vi "LCR_Readout.vi"(8 "error in (no error)":errorcluster, 11 "WK6440B in":refnum<class "WK6440B.lvclass">) -> (0 "error out":errorcluster, 1 "Resistance in Ohm":dbl, 2 "Capacitance in pF":dbl, 3 "WK6440B out":refnum<class "WK6440B.lvclass">)   [LabVIEW 2018, in "WK6440B.lvclass"]
uses:
  WK6440B.lvclass
  F:/itk-strip-sensor-qc/LabVIEW 2013/InstrControl/InstrControl.lvclass
  InstrControl.lvclass
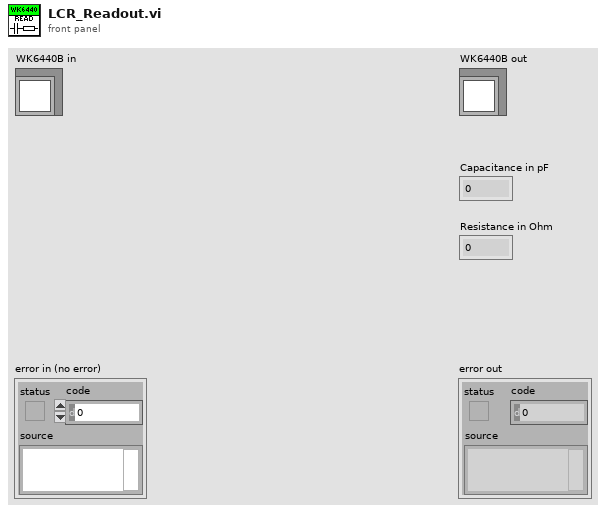
[diagram p1: front panel]
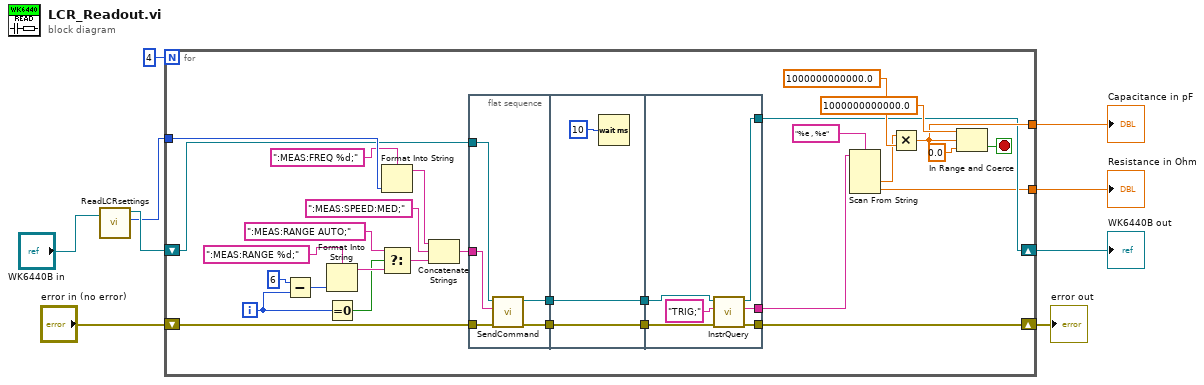
[diagram p0: block diagram]
diagram:
  n1 = call-dynamic "ReadLCRsettings.vi"("LCRControl in"="WK6440B in") -> ("AC frequency [Hz]"=w1:i32, "LCRControl out"=w2:refnum<class "WK6440B.lvclass">)  [unwired: 1 in, 3 out]
  n2 = for {
    N: 4 -> [_]
    tunnel: [w10] -> w5
    tunnel: [w36] -> w6
    tunnel: w1 -> [w33]
    shift-right: [w11] -> w4
    shift-left: w2 -> [w18]
    shift-right: [w16] -> w7
    shift-left: "error in (no error)" -> [w32]
    i -> [w35]
    stop <- w34 stop-if-true
    n3 = Subtract(x=6, y=w35) -> (x-y=w22:i32)
    n4 = Format Into String(format string=":MEAS:RANGE %d;", w22) -> (resulting string=w25:string)  [unwired: 2 in, 1 out]
    n5 = Equal To 0?(x=w35) -> (x = 0?=w24:bool)
    n6 = Format Into String(format string=":MEAS:FREQ %d;", w33) -> (resulting string=w31:string)  [unwired: 2 in, 1 out]
    n7 = Select(t=":MEAS:RANGE AUTO;", s=w24, f=w25) -> (s? t:f=w28:string)
    n8 = Concatenate Strings(w31, ":MEAS:SPEED:MED;", w28) -> (w39:string)
    n9 = flat-sequence {
      tunnel: w39 -> [w42]
      tunnel: w32 -> [w44]
      tunnel: w18 -> [w40]
      tunnel: [w43] -> w15
      tunnel: [w41] -> w13
      tunnel: w15 -> [w46]
      tunnel: [w46] -> w14
      tunnel: w13 -> [w45]
      tunnel: [w45] -> w12
      tunnel: [w52] -> w16
      tunnel: [w51] -> w17
      tunnel: w14 -> [w53]
      tunnel: w12 -> [w49]
      tunnel: [w48] -> w11
      frame #0 {
        n10 = call "SendCommand.vi"("error in (no error)"=w44, "Command string"=w42, "InstControl in"=w40) -> ("error out"=w43:errorcluster, "InstControl out"=w41:refnum<class "WK6440B.lvclass">)  [unwired: 7 in]
      }
      frame #1 {
        n11 = Wait (ms)(milliseconds to wait=10) -> ()  [unwired: 1 out]
      }
      frame #2 {
        n12 = call-dynamic "InstrQuery.vi"("error in (no error)"=w53, "Command string"="TRIG;", "InstControl in"=w49) -> ("error out"=w52:errorcluster, "Instrument response"=w51:string, "InstControl out"=w48:refnum<class "WK6440B.lvclass">)  [unwired: 6 in]
      }
    }
    n13 = Scan From String(format string="%e , %e", input string=w17) -> (output 1=w19:dbl, output 2=w10:dbl)  [unwired: 4 in, 3 out]
    n14 = Multiply(x=w19, y=1000000000000.0) -> (x*y=w36:dbl)
    n15 = In Range and Coerce(upper limit=1000000000000.0 ("y"), x=w36, lower limit=0.0) -> (In Range?=w34:bool)  [unwired: 1 out]
  }
  "error out" <- w7
  "WK6440B out" <- w4
  "Capacitance in pF" <- w6
  "Resistance in Ohm" <- w5
